vi "saveControls.vi"(7 "prevName":string caption="default name", 8 "error in (no error)":errorcluster, 9 "isAutoSave":bool, 10 "ConfigXMLControls":T1, 11 "ControlsToSave":refnum<vi>[](array[refnum])) -> (0 "error out":errorcluster, 3 "nameUsed":string caption="default name")   [LabVIEW 2016]
uses:
  ConfigXMLControl.ctl
  General/CorePluginInfo.ctl
panel:
  # "Saves the selected controls to an XML file. This will save an XML file\nin the selected directory named ConfigName, or prompt the user for\na name if it is blank. In autosave mode, this saves it into the autosave\ndirectory, in a subdirectory for the current date, and named after the \ncurrent timestamp."
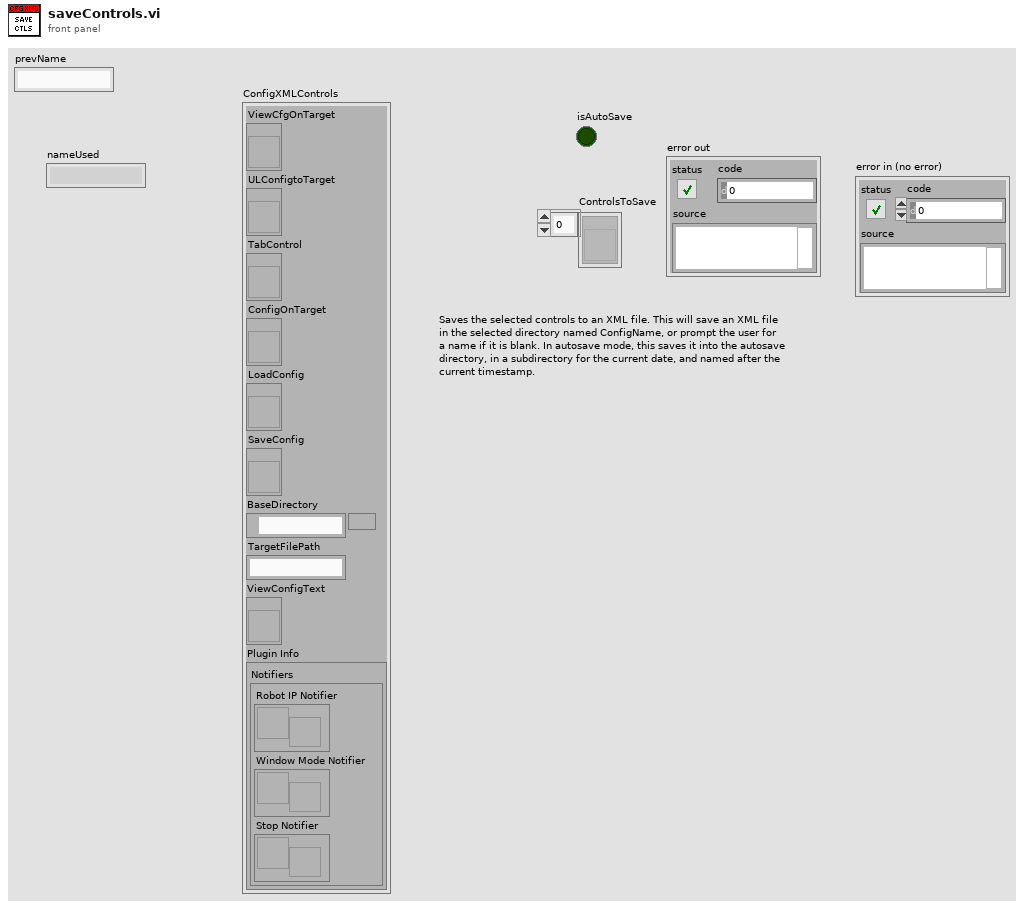
[diagram p1: front panel]
types:
  T1 = typedef "ConfigXMLControl.ctl" = cluster{"ViewCfgOnTarget":refnum<vi>, "ULConfigtoTarget":refnum<vi>, "TabControl":refnum<vi>, "ConfigOnTarget":refnum<vi>, "LoadConfig":refnum<vi>, "SaveConfig":refnum<vi>, "BaseDirectory":path, "TargetFilePath":string, "ViewConfigText":refnum<vi>, "Plugin Info":T2}
  T2 = typedef "CorePluginInfo.ctl" = cluster{"Notifiers":cluster{"Robot IP Notifier":refnum<notifier>, "Window Mode Notifier":refnum<notifier>, "Stop Notifier":refnum<notifier>}}
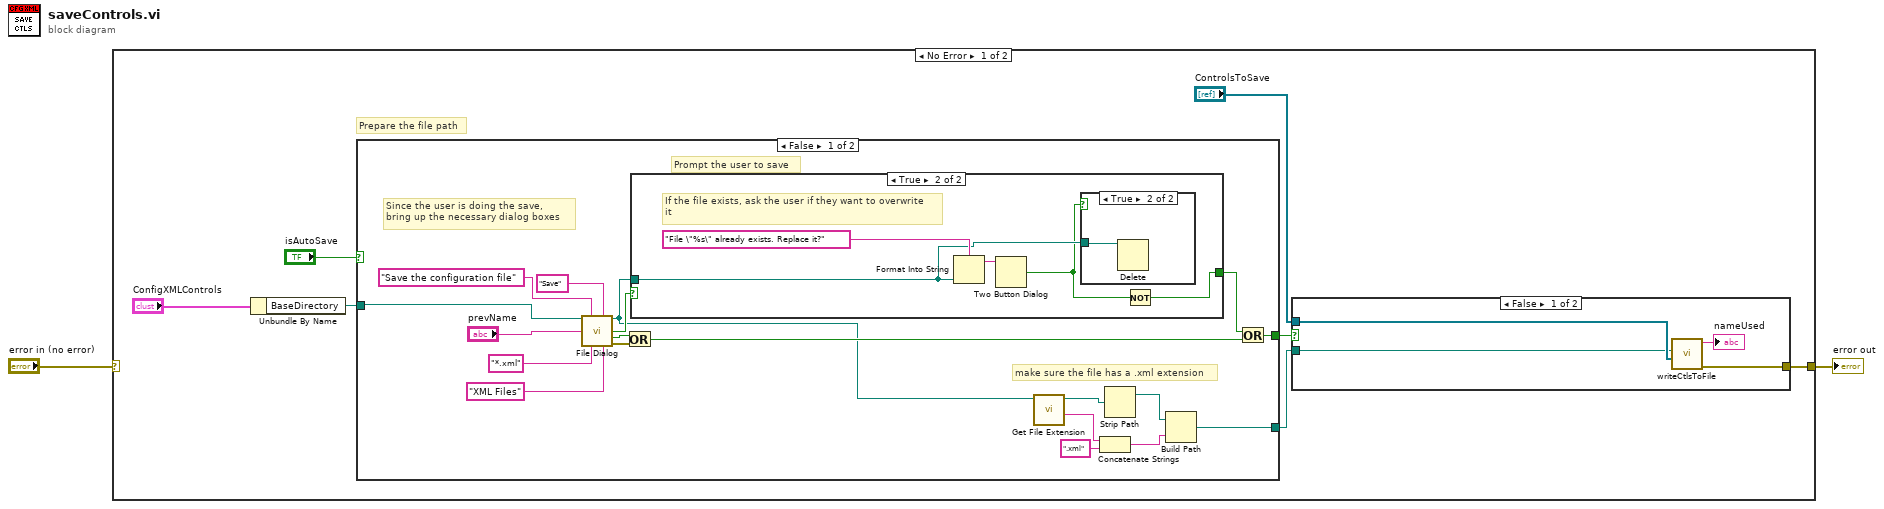
[diagram p0: block diagram]
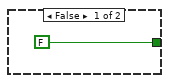
[diagram p3: hidden frame]
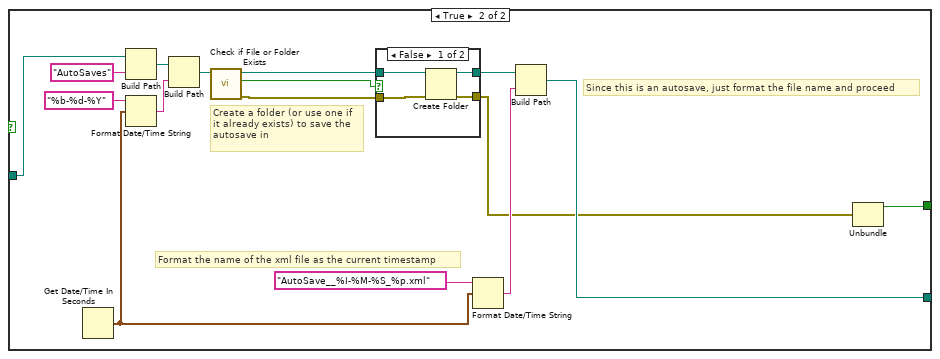
[diagram p5: hidden frame]
diagram:
  n1 = case shown="No Error" "error in (no error)" {
    selector: "error in (no error)" -> [_ w61]
    tunnel: [w3 w61] -> w2
    frame No Error {
      # "Prepare the file path"
      n2 = Unbundle By Name("ConfigXMLControls") -> ("BaseDirectory"=w7:path)
      n3 = case shown="False" "isAutoSave" {
        tunnel: w7 -> [w15 w43]
        tunnel: [w14 w40] -> w6
        tunnel: [w16 w44] -> w5
        frame False {
          # "make sure the file has a .xml extension"
          # "Since the user is doing the save, \nbring up the necessary dialog boxes"
          # "Prompt the user to save"
          n4 = call "File Dialog"("start path"=w15, "prompt"="Save the configuration file", "button label"="Save", "default name"="prevName", "pattern (all files)"="*.xml", "pattern label"="XML Files") -> ("selected path"=w22:path, "exists"=w28:bool, "cancelled"=w27:bool, "error out"=w26:errorcluster)  [unwired: 6 in]
          n5 = Or(x=w27, y=w26) -> (x .or. y?=w24:bool)
          n6 = case shown="True" w28 {
            tunnel: w22 -> [_ w36]
            tunnel: [FALSE ("T button?") w34] -> w25
            frame False {
            }
            frame True {
              # "If the file exists, ask the user if they want to overwrite\nit"
              n7 = Format Into String(format string="File \"%s\" already exists. Replace it?", w36) -> (resulting string=w37:string)  [unwired: 2 in, 1 out]
              n8 = Two Button Dialog(message=w37) -> (T button?=w35:bool)  [unwired: 2 in]
              n9 = case shown="True" w35 {
                tunnel: w36 -> [_ w39]
                frame False {
                }
                frame True {
                  n10 = Delete(path (use dialog)=w39) -> ()  [unwired: 4 in, 3 out]
                }
              }
              n11 = Not(x=w35) -> (.not. x?=w34:bool)
            }
          }
          n12 = call <vilib>:"Get File Extension.vi"("file"=w22) -> ("filename without extension"=w20:string, "dup file"=w21:path)  [unwired: 6 in, 3 out]
          n13 = Concatenate Strings(w20, ".xml" ("string")) -> (w17:string)
          n14 = Strip Path(path=w21) -> (stripped path=w18:path)  [unwired: 1 out]
          n15 = Build Path(base path=w18, name or relative path=w17) -> (appended path=w16:path)
          n16 = Or(x=w25, y=w24) -> (x .or. y?=w14:bool)
        }
        frame True {
          # "Format the name of the xml file as the current timestamp"
          # "Create a folder (or use one if\nit already exists) to save the\nautosave in"
          # "Since this is an autosave, just format the file name and proceed"
          n17 = Get Date/Time In Seconds() -> (seconds since 1Jan1904=w53:timestamp)
          n18 = Build Path(base path=w43, name or relative path="AutoSaves") -> (appended path=w51:path)
          n19 = Format Date/Time String(time format string (%c)="%b-%d-%Y", seconds (now)=w53) -> (date/time string=w50:string)  [unwired: 1 in]
          n20 = Build Path(base path=w51, name or relative path=w50) -> (appended path=w49:path)
          n21 = call <vilib>:"Check if File or Folder Exists.vi"("path"=w49) -> ("error out"=w42:errorcluster, "file or folder exists?"=w48:bool, "dup path"=w47:path)  [unwired: 8 in]
          n22 = case shown="False" w48 {
            tunnel: w47 -> [w59 w60]
            tunnel: [w58 w60] -> w46
            tunnel: [w57 _] -> w41
            tunnel: w42 -> [w56 _]
            frame False {
              n23 = Create Folder(path (use dialog)=w59, error in=w56) -> (created path=w58:path, error out=w57:errorcluster)  [unwired: 1 in, 1 out]
            }
            frame True {
            }
          }
          n24 = Format Date/Time String(time format string (%c)="AutoSave__%I-%M-%S_%p.xml", seconds (now)=w53) -> (date/time string=w45:string)  [unwired: 1 in]
          n25 = Build Path(base path=w46, name or relative path=w45) -> (appended path=w44:path)
          n26 = Unbundle(w41) -> ("status"=w40:bool)  [unwired: 2 out]
        }
      }
      n27 = case shown="False" w6 {
        tunnel: w5 -> [w11 _]
        tunnel: "ControlsToSave" -> [w13 _]
        tunnel: [w12 _] -> w3
        frame False {
          n28 = call "writeCtlsToFile.vi"("ControlsToSave"=w13, "path"=w11) -> ("error out"=w12:errorcluster, "nameUsed"=→"nameUsed":string)  [unwired: 8 in]
        }
        frame True {
          # "If true, then the save was either declined by the user, or there was some other error,\nso do not save the file"
        }
      }
    }
    frame Error {
    }
  }
  "error out" <- w2
